vi "ActionVIOnCompile.vi"(8 "error in (no error)":errorcluster, 11 "Device Item Ref in":T1 format="%.0x") -> (0 "error out":errorcluster)   [LabVIEW 2015, in "Waveform-Processing-Custom-Device System Explorer.lvlib"]
uses:
  Waveform-Processing-Custom-Device System Explorer.lvlib
  <vilib>/NI Veristand/Custom Device API/Custom Device Item Ref.ctl
  Shared/Types/FG Action.ctl
  Shared/CompiledSettings.ctl
  <vilib>/NI Veristand/Custom Device API/Block Data Reference.ctl
  <vilib>/NI Veristand/Custom Device API/Data Reference.ctl
  <vilib>/NI Veristand/Custom Device API/Waveform Data Reference.ctl
  Shared/Constants.vi
  <vilib>/NI Veristand/Custom Device API/Set Item Property (Variant).vi
  <vilib>/NI VeriStand/Custom Device API/Custom Device API.lvlib
  <vilib>/NI/NIVS Inline Async API/_Data Access System Explorer/Data Access System Explorer.lvlib
  Shared/Waveform-Processing-Custom-Device Shared.lvlib
  Shared/Running Average/Running Average.lvlib
  Shared/Single Point/SinglePoint.lvlib
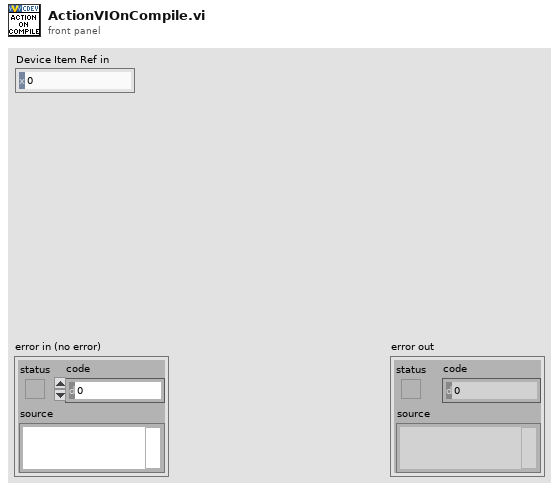
[diagram p1: front panel]
types:
  T1 = typedef "Custom Device API.lvlib/Custom Device Item Ref.ctl" = u64
  T2 = typedef "Waveform-Processing-Custom-Device Shared.lvlib/CompiledSettings.ctl" = cluster{"Name":string, "Buffer Length (samples)":u32, "Enable Array":bool[], "Parameter Block Data Refs":T3[], "Source Wfm Data Refs":T5[], "Result Wfm Data Refs":T5[], "Result Ch Data Refs":T4[], "Task Rate (Hz)":dbl}
  T3 = typedef "Custom Device API.lvlib/Block Data Reference.ctl" = cluster{"Data Reference":T4, "Offset":u64, "Length":u64}
  T4 = typedef "Custom Device API.lvlib/Data Reference.ctl" = i32
  T5 = typedef "Custom Device API.lvlib/Waveform Data Reference.ctl" = i32
  T6 = typedef "Waveform-Processing-Custom-Device Shared.lvlib/FG Action.ctl" = enum8{"GET", "SET"}
  T7 = typedef "Custom Device API.lvlib/Custom Device Item Info.ctl" = cluster{"Name":string, "Is Channel":bool, "GUID":string, "Is Waveform":bool}
  T8 = typedef "Waveform-Processing-Custom-Device Shared.lvlib/Custom Device Settings.ctl" = cluster{"CD Task Dependency":T1, "CD Task Dependency Ref":T1, "CD Task Available Wfms":string[], "CD Task Selected Wfms":string[], "Buffer Length (s)":dbl, "Buffer Length (samples)":u32, "Single-point Enabled":bool, "Running Average Enabled":bool, "Task Rate":dbl}
  T9 = cluster{"Name":string, "Type":enum16{"Output/Write", "Input/Read", "Input/ReadWrite"}, "VS Refs":T1[]}[]
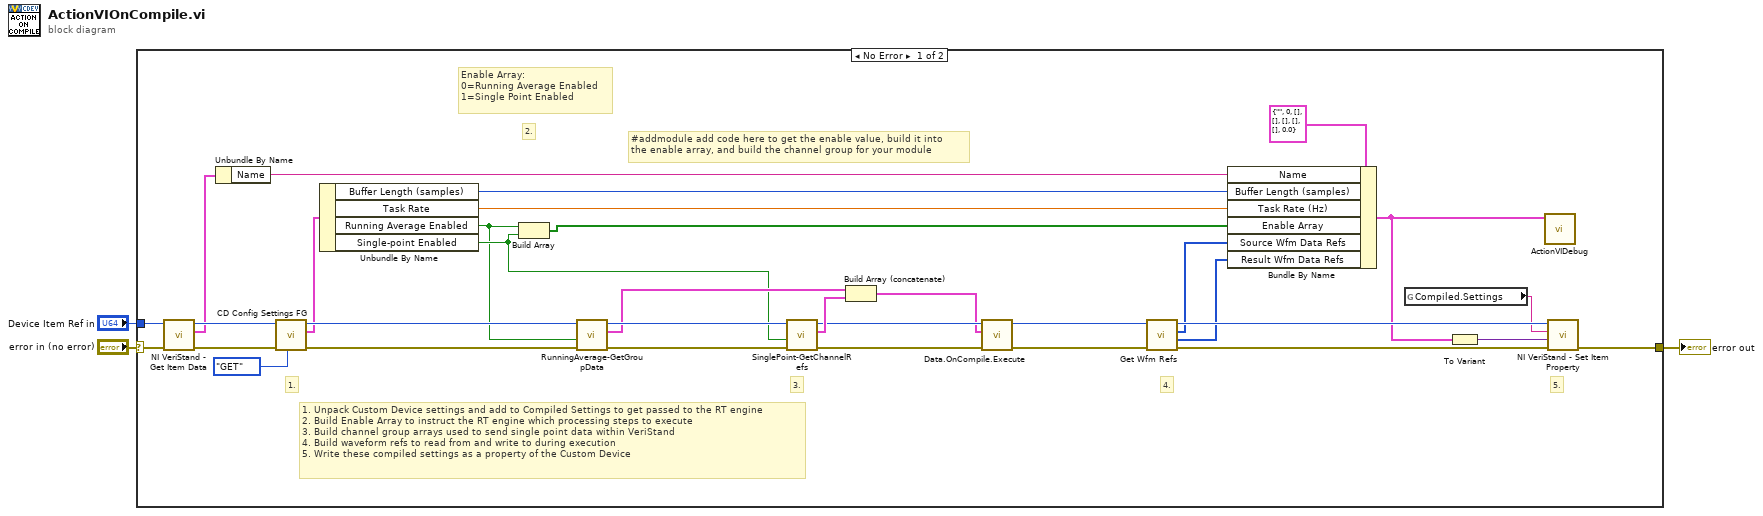
[diagram p0: block diagram]
diagram:
  n1 = case shown="No Error" "error in (no error)" {
    selector: "error in (no error)" -> [w35 w37]
    tunnel: [w36 w37] -> w2
    tunnel: "Device Item Ref in" -> [w34 _]
    frame No Error {
      # "#addmodule add code here to get the enable value, build it into\nthe enable array, and build the channel group for your module"
      # "Enable Array:\n0=Running Average Enabled\n1=Single Point Enabled"
      # "5."
      # "4."
      # "3."
      # "2."
      # "1."
      # "1. Unpack Custom Device settings and add to Compiled Settings to get passed to the RT engine\n2. Build Enable Array to instruct the RT engine which processing steps to execute\n3. Build channel group arrays used to send single point data within VeriStand\n4. Build waveform refs to read from and write to during execution\n5. Write these compiled settings as a property of the Custom Device"
      n2 = call <vilib>:"NI VeriStand - Get Item Data.vi"("error in (no error)"=w35, "Item Ref in"=w34) -> ("error out"=w32:errorcluster, "Item Info"=w31:T7, "Item Ref out"=w33:T1)  [unwired: 6 in, 1 out]
      n3 = Unbundle By Name(w31) -> ("Name"=w21:string)
      n4 = call "CD Config Settings FG.vi"("Action"=FG_Action."GET", "error in (no error)"=w32, "Item Ref"=w33) -> ("error out"=w29:errorcluster, "CD Settings out"=w20:T8, "Item Ref out"=w24:T1)  [unwired: 5 in, 1 out]
      n5 = Unbundle By Name(w20) -> ("Buffer Length (samples)"=w19:u32, "Task Rate"=w8:dbl, "Running Average Enabled"=w10:bool, "Single-point Enabled"=w11:bool)
      n6 = Build Array(w10, w11) -> (w9:bool[])
      n7 = call "RunningAverage-GetGroupData.vi"("Error in"=w29, "Enabled?"=w10, "Device Ref in"=w24) -> ("Error out"=w28:errorcluster, "Group Data Array"=w18:T9, "Device Ref out"=w23:T1)  [unwired: 6 in]
      n8 = call "SinglePoint-GetChannelRefs.vi"("Error in"=w28, "Enabled?"=w11, "Device Ref in"=w23) -> ("Error out"=w14:errorcluster, "Group Data Array"=w17:T9, "Device Ref out"=w16:T1)  [unwired: 6 in]
      n9 = Build Array (concatenate)(w18, w17) -> (w12:T9)
      n10 = call <vilib>:"Data.OnCompile.Execute.vi"("error in"=w14, "VS Ref Groups"=w12, "Custom Device Ref"=w16) -> ("error out"=w13:errorcluster, "Custom Device Ref"=w15:T1)  [unwired: 7 in]
      n11 = call "Get Wfm Refs.vi"("Error in"=w13, "Device Ref in"=w15) -> ("Error out"=w27:errorcluster, "Results Wfm Data Refs"=w6:T5[], "Source Wfm Data Refs"=w7:T5[], "Device Ref out"=w22:T1)  [unwired: 6 in]
      n12 = Bundle By Name(cluster=T2 {"Name"="", "Buffer Length (samples)"=0, "Enable Array"=[], "Parameter Block Data Refs"=[], "Source Wfm Data Refs"=[], "Result Wfm Data Refs"=[], "Result Ch Data Refs"=[], "Task Rate (Hz)"=0.0} ("CompiledSettings"), "Name"=w21, "Buffer Length (samples)"=w19, "Task Rate (Hz)"=w8, "Enable Array"=w9, "Source Wfm Data Refs"=w7, "Result Wfm Data Refs"=w6) -> (w4:T2)
      n13 = global read "Constants.vi" "Compiled.Settings"() -> (w5:string)
      n14 = To Variant(anything=w4) -> (Variant=w25:variant)
      n15 = call "ActionVIDebug.vi"("CompiledSettings"=w4) -> ()  [unwired: 11 in]
      n16 = call-poly <vilib>:"NI VeriStand - Set Item Property.vi"("error in (no error)"=w27, "Value"=w25, "Property Name"=w5, "Item Ref in"=w22) -> ("error out"=w36:errorcluster)  [unwired: 5 in, 2 out]
    }
    frame Error {
    }
  }
  "error out" <- w2
